vi "Get 经度.vi"(11 "GPS in":refnum<class "GPS.lvclass">) -> (2 "经度":refnum<vi>, 3 "GPS out":refnum<class "GPS.lvclass">)   [LabVIEW 2016, in "GPS.lvlib" / "GPS.lvclass"]
uses:
  GPS.lvclass
  GPS.lvclass/GPS.ctl
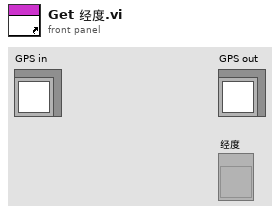
[diagram p1: front panel]
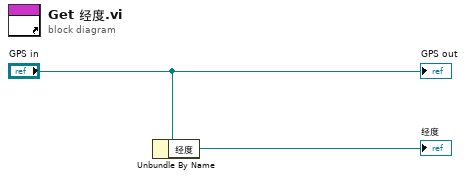
[diagram p0: block diagram]
diagram:
  n1 = Unbundle By Name("GPS in") -> ("经度"=→"经度":refnum<vi>)
  "GPS out" <- "GPS in"
